vi "BackupDB.vi"(8 "error in (no error)":errorcluster, 11 "object in":refnum<class "TableLogger_Actor.lvclass">) -> (0 "error out":errorcluster, 3 "object out":refnum<class "TableLogger_Actor.lvclass">)   [LabVIEW 2014, in "TableLogger_Actor.lvlib" / "TableLogger_Actor.lvclass"]
uses:
  TableLogger_Actor.lvclass
  TableLogger_Actor.lvclass/TableLogger_Actor.ctl
panel:
  # "Connector Pane"
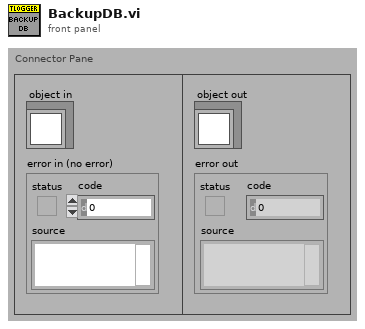
[diagram p1: front panel]
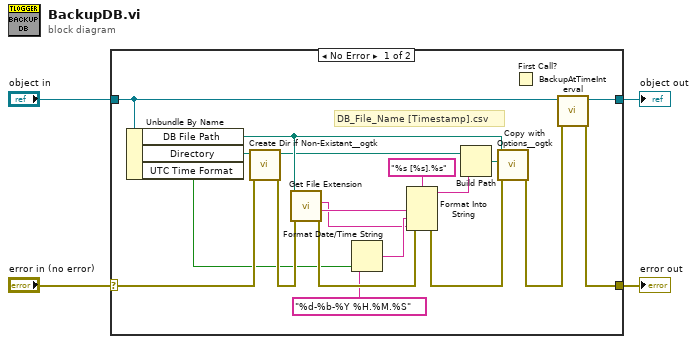
[diagram p0: block diagram]
diagram:
  n1 = case shown="No Error" "error in (no error)" {
    selector: "error in (no error)" -> [w13 w25]
    tunnel: [w7 w25] -> w3
    tunnel: [w9 w24] -> w1
    tunnel: "object in" -> [w10 w24]
    frame No Error {
      # "DB_File_Name [Timestamp].csv"
      n2 = Unbundle By Name(w10) -> ("DB File Path"=w23:path, "Directory"=w22:path, "UTC Time Format"=w6:bool)
      n3 = call <userlib>:"Create Dir if Non-Existant__ogtk.vi"("error in (no error)"=w13, "Directory Path"=w22) -> ("error out"=w19:errorcluster, "dup Directory Path"=w18:path)  [unwired: 7 in, 1 out]
      n4 = call <vilib>:"Get File Extension.vi"("error in (no error)"=w19, "file"=w23) -> ("error out"=w20:errorcluster, "filename without extension"=w16:string, "lowercase file extension"=w5:string)  [unwired: 6 in, 1 out]
      n5 = Format Date/Time String(time format string (%c)="%d-%b-%Y %H.%M.%S", UTC format=w6) -> (date/time string=w11:string)  [unwired: 1 in]
      n6 = Format Into String(format string="%s [%s].%s", error in=w20, w16, w11, w5) -> (resulting string=w15:string, error out=w14:errorcluster)  [unwired: 1 in]
      n7 = Build Path(base path=w18, name or relative path=w15) -> (appended path=w21:path)
      n8 = call <userlib>:"Copy with Options__ogtk.vi"("error in (no error)"=w14, "target path"=w21, "source path"=w23) -> ("error out"=w8:errorcluster)  [unwired: 7 in, 1 out]
      n9 = First Call?() -> ()  [unwired: 1 out]
      n10 = call "BackupAtTimeInterval.vi"("error in (no error)"=w8, "object in"=w10) -> ("error out"=w7:errorcluster, "object out"=w9:refnum<class "TableLogger_Actor.lvclass">)  [unwired: 8 in]
    }
    frame Error {
    }
  }
  "error out" <- w3
  "object out" <- w1
